vi "Select a Path.vi"(9 "Display State In":T2 caption="显示状态输入", 11 "Include Paths Ref":refnum<vi> caption="包括路径引用") -> (1 "Display State Out":T2 caption="显示状态输出", 2 "Path Strings Out":T1 caption="路径字符串输出", 3 "Dup Include Paths Ref":refnum<vi> caption="包括路径引用副本", 4 "cancelled":bool caption="取消")   [LabVIEW 2012, in "NISAST Include Paths.xctl"]
uses:
  NISAST Include Paths.xctl
  State.ctl
  Data.ctl
  Instance           1 21Saved   Select a Path .vi
panel:
  in  "prompt":string="选择包括路径" caption="提示"
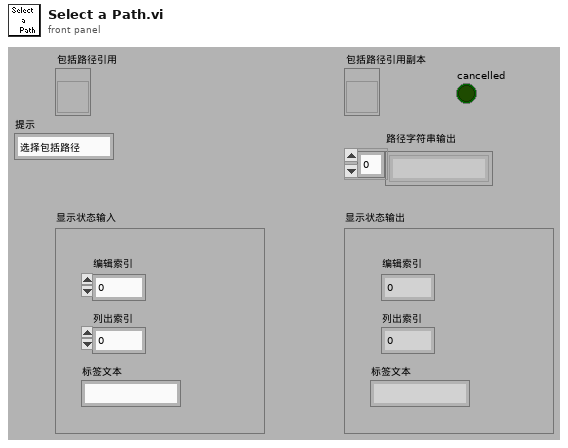
[diagram p1: front panel]
types:
  T1 = typedef "NISAST Include Paths.xctl/Data.ctl" = string[]
  T2 = typedef "NISAST Include Paths.xctl/State.ctl" = cluster{"Edit Index":i32, "List Index":i32, "Label Text":string}
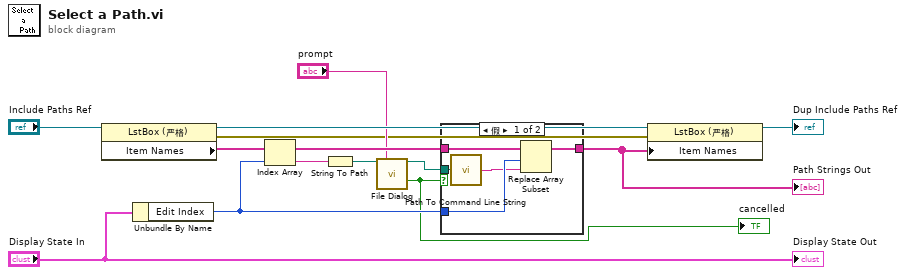
[diagram p0: block diagram]
diagram:
  n1 = property class="LstBox (严格)"(reference="Include Paths Ref") -> (reference out=w8:refnum<vi>, error out=w5:errorcluster, "Item Names"=w9:string[])  [unwired: 1 in]
  n2 = Unbundle By Name("Display State In") -> ("Edit Index"=w4:i32)
  n3 = Index Array(array=w9, index=w4) -> (element=w12:string)
  n4 = String To Path(string=w12) -> (path=w13:path)
  n5 = call "File Dialog"("start path"=w13, "prompt"="prompt") -> ("selected path"=w10:path, "cancelled"=w1:bool)  [unwired: 10 in, 2 out]
  "cancelled" <- w1
  n6 = case shown="假" w1 {
    tunnel: w10 -> [w15 _]
    tunnel: w9 -> [w18 w19]
    tunnel: w4 -> [w17 _]
    tunnel: [w16 w19] -> w2
    frame False {
      n7 = call <vilib>:"Path To Command Line String.vi"("path"=w15) -> ("string"=w14:string)
      n8 = Replace Array Subset(array=w18, new element=w14, index=w17) -> (w16:string[])
    }
    frame True {
    }
  }
  "Path Strings Out" <- w2
  n9 = property class="LstBox (严格)"(reference=w8, error in=w5, "Item Names"=w2) -> (reference out=→"Dup Include Paths Ref":refnum<vi>)  [unwired: 1 out]
  "Display State Out" <- "Display State In"
